vi "Start Sync.vi"(8 "error in (no error)":errorcluster, 11 "gRPC Server in":refnum<class "Data Marshal Server.lvclass">) -> (0 "error out":errorcluster, 3 "gRPC Server out":refnum<class "Data Marshal Server.lvclass">)   [LabVIEW 2019, in "Data Marshal Server.lvlib" / "Data Marshal Server.lvclass"]
uses:
  Data Marshal Server.lvclass
  RPC Messages/TestDataTypesParameters/TestDataTypesParameters_Data.ctl
  RPC Messages/DataTypeTest/DataTypeTest_Data.ctl
  gRPC lvSupport/Server API/typeDefs/grpcId.ctl
  Data Marshal Server.lvclass/Data Marshal Server.ctl
  RPC Messages/ServerEvent/ServerEvent_Data.ctl
  RPC Messages/InvokeResponse/InvokeResponse_Data.ctl
  RPC Messages/QueryResponse/QueryResponse_Data.ctl
  gRPC lvSupport/gprc-lvsupport.lvlib
panel:
  out "Message Data":T1
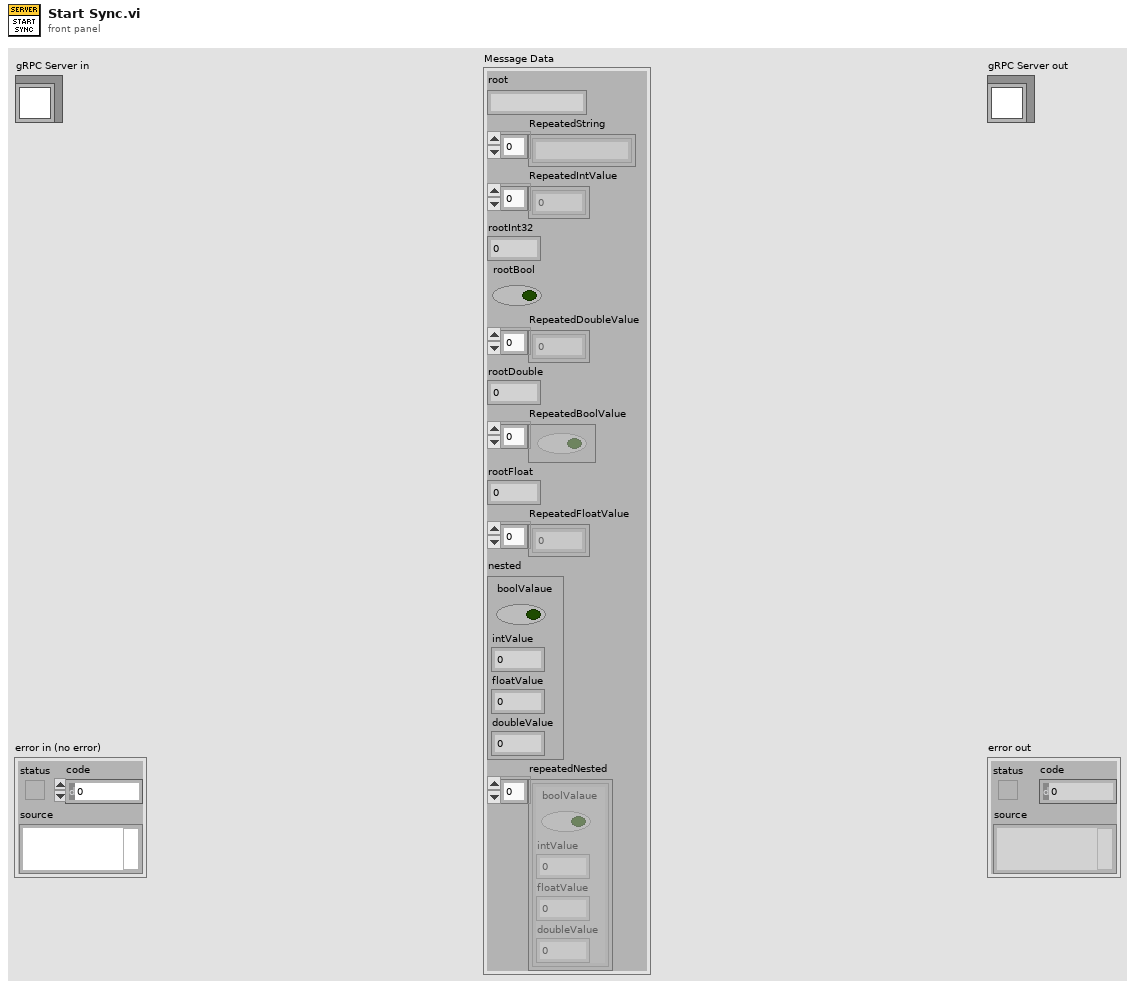
[diagram p1: front panel]
types:
  T1 = typedef "Data Marshal Server.lvlib/Data Marshal Server.lvclass/TestDataTypesParameters_Data.ctl" = cluster{"root":string, "RepeatedString":string[], "RepeatedIntValue":i32[], "rootInt32":i32, "rootBool":bool, "RepeatedDoubleValue":dbl[], "rootDouble":dbl, "RepeatedBoolValue":bool[], "rootFloat":sgl, "RepeatedFloatValue":sgl[], "nested":T2, "repeatedNested":T2[]}
  T2 = typedef "Data Marshal Server.lvlib/Data Marshal Server.lvclass/DataTypeTest_Data.ctl" = cluster{"boolValaue":bool, "intValue":i32, "floatValue":sgl, "doubleValue":dbl}
  T3 = typedef "Data Marshal Server.lvlib/gprc-lvsupport.lvlib/grpcId.ctl" = u64
  T4 = typedef "Data Marshal Server.lvlib/Data Marshal Server.lvclass/ServerEvent_Data.ctl" = cluster{"eventData":string, "serverId":i32, "status":i32}
  T5 = typedef "Data Marshal Server.lvlib/Data Marshal Server.lvclass/InvokeResponse_Data.ctl" = cluster{"status":i32}
  T6 = typedef "Data Marshal Server.lvlib/Data Marshal Server.lvclass/QueryResponse_Data.ctl" = cluster{"message":string, "status":i32}
  T7 = typedef "Data Marshal Server.lvlib/Data Marshal Server.lvclass/Server gRPC UEs.ctl" = cluster{"Invoke gRPC UE":refnum<user-event>, "Query gRPC UE":refnum<user-event>, "Register gRPC UE":refnum<user-event>, "TestDataTypes gRPC UE":refnum<user-event>}
  T8 = typedef "Data Marshal Server.lvlib/Data Marshal Server.lvclass/InvokeRequest_Data.ctl" = cluster{"command":string, "parameter":string}
  T9 = typedef "Data Marshal Server.lvlib/Data Marshal Server.lvclass/QueryRequest_Data.ctl" = cluster{"query":string}
  T10 = typedef "Data Marshal Server.lvlib/Data Marshal Server.lvclass/RegistrationRequest_Data.ctl" = cluster{"eventName":string}
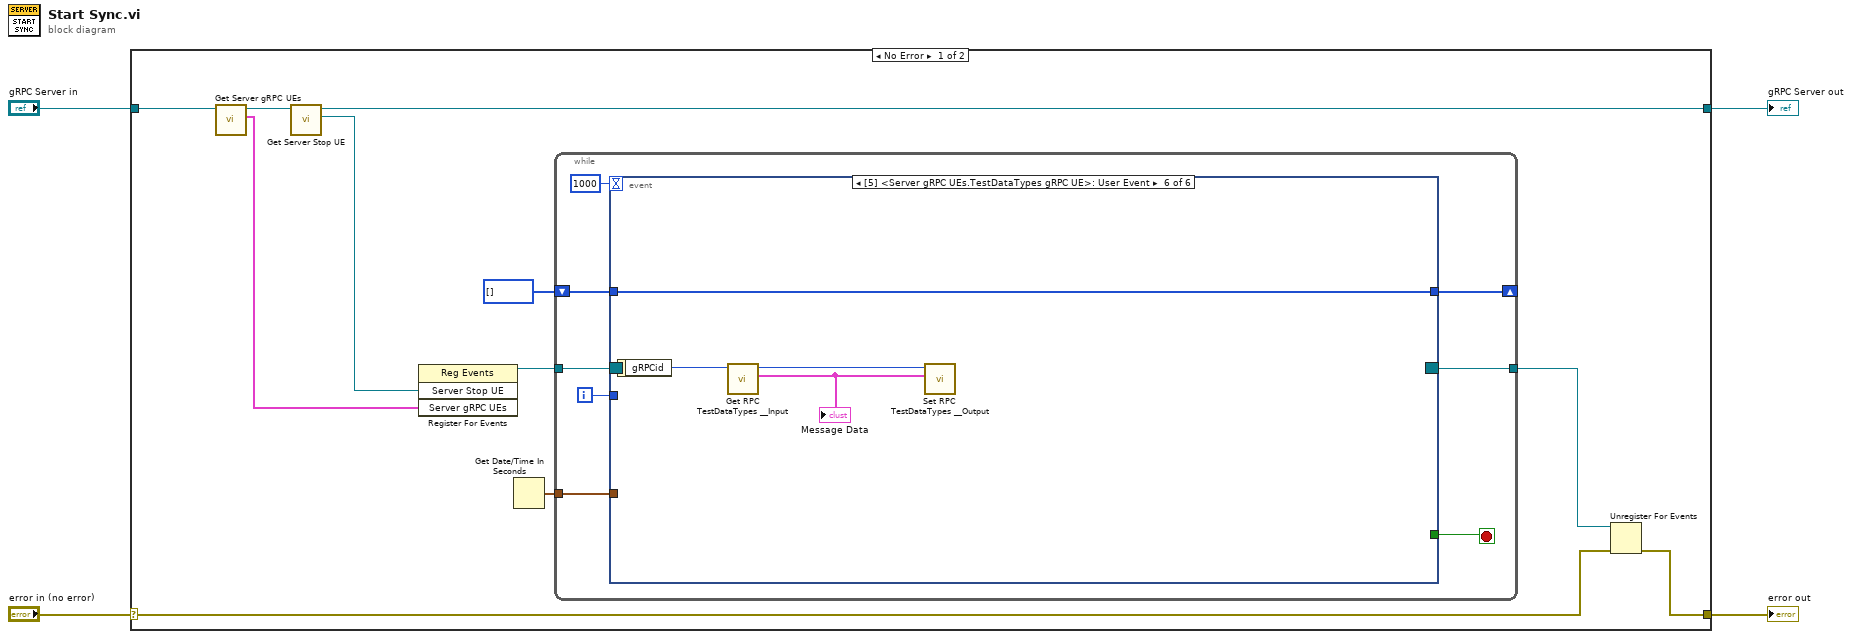
[diagram p0: block diagram]
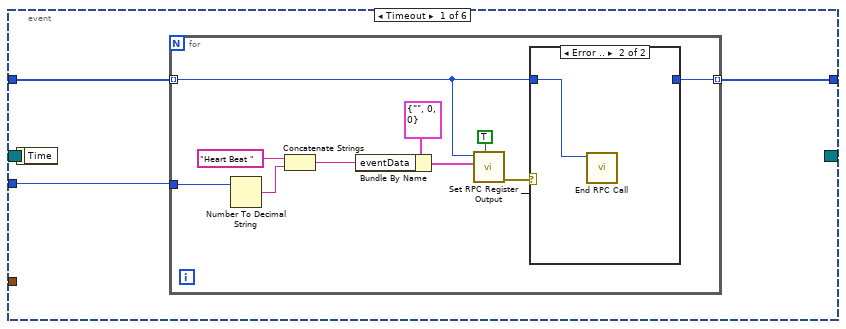
[diagram p2: hidden frame]
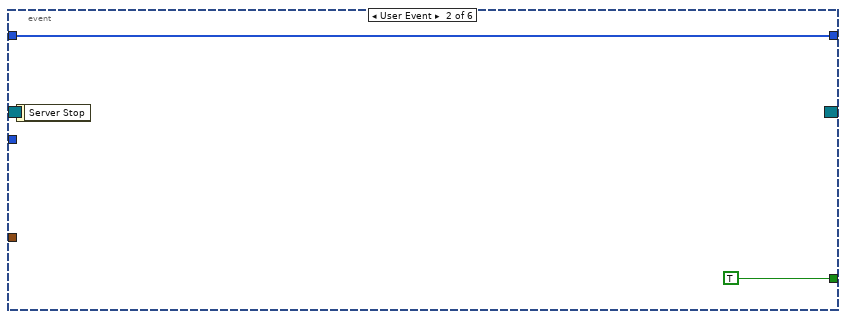
[diagram p4: hidden frame]
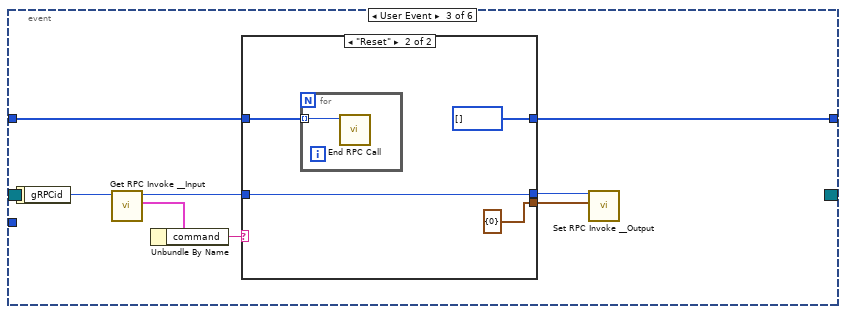
[diagram p5: hidden frame]
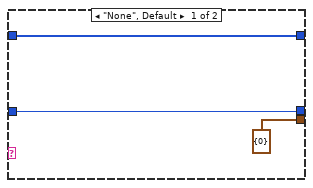
[diagram p6: hidden frame]
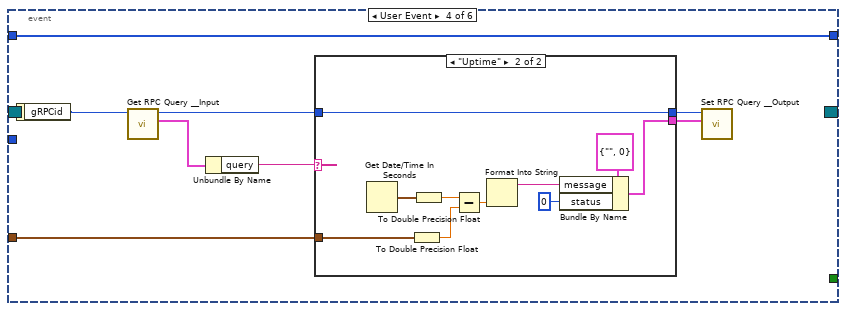
[diagram p7: hidden frame]
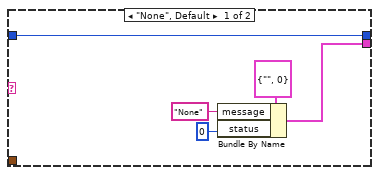
[diagram p8: hidden frame]
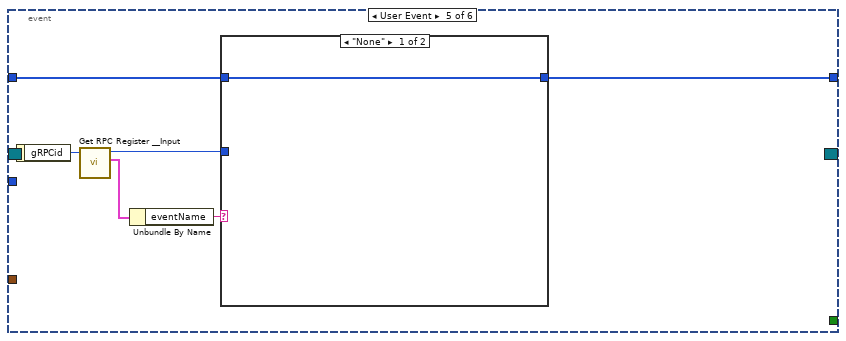
[diagram p9: hidden frame]
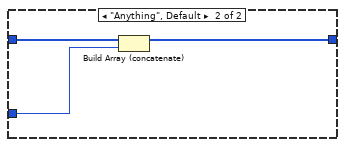
[diagram p10: hidden frame]
diagram:
  n1 = case shown="No Error" "error in (no error)" {
    selector: "error in (no error)" -> [w8 w95]
    tunnel: [w7 w95] -> w3
    tunnel: [w11 w94] -> w1
    tunnel: "gRPC Server in" -> [w15 w94]
    frame No Error {
      n2 = call "Get Server gRPC UEs.vi"("OOP Server in"=w15) -> ("Server gRPC UEs"=w12:T7, "OOP Server out"=w14:refnum<class "Data Marshal Server.lvclass">)  [unwired: 9 in]
      n3 = call "Get Server Stop UE.vi"("OOP Server in"=w14) -> ("Server Stop UE"=w13:refnum<user-event>, "OOP Server out"=w11:refnum<class "Data Marshal Server.lvclass">)  [unwired: 9 in]
      n4 = register-events(w13, w12) -> (reference out=w10:refnum<event-registration>)  [unwired: 2 in, 1 out]
      n5 = Get Date/Time In Seconds() -> (seconds since 1Jan1904=w5:timestamp)
      n6 = while {
        tunnel: w10 -> [w23]
        tunnel: [w21] -> w9
        shift-right: [w18] -> _
        shift-left: T3[] [] ("appended array") -> [w19]
        tunnel: w5 -> [w16]
        i -> [w17]
        stop <- w22 stop-if-true
        n7 = event "RPC Methods Event Structure" shown="[5] <Server gRPC UEs.TestDataTypes gRPC UE>: User Event" {
          selector: w23 -> [_ _ _ _ _ _]
          dyn-events: [_ _ _ _ _ _] -> w21
          timeout: 1000 -> [_ _ _ _ _ _]
          tunnel: [_ TRUE _ _ _ _] -> w22
          tunnel: w19 -> [w26 w39 w45 w64 w81 w93]
          tunnel: [w25 w39 w44 w64 w80 w93] -> w18
          tunnel: w17 -> [w24 _ _ _ _ _]
          tunnel: w16 -> [_ _ _ w57 _ _]
          event Timeout {
            n8 = event-data() -> ()  [unwired: 1 in, 1 out]
            n9 = for {
              tunnel: w26 -> [w29] mode=indexing
              tunnel: w24 -> [w33]
              tunnel: [w27] -> w25 mode=indexing
              n10 = Number To Decimal String(number=w33) -> (decimal integer string=w36:string)  [unwired: 1 in]
              n11 = Concatenate Strings("Heart Beat " ("eventdata"), w36) -> (w34:string)
              n12 = Bundle By Name(cluster=T4 {"eventData"="", "serverId"=0, "status"=0} ("Message Data"), "eventData"=w34) -> (w30:T4)
              n13 = call "Set RPC Register __Output.vi"("Streeming? (F)"=TRUE, "Message Data"=w30, "gRPCid in"=w29) -> ("error out"=w28:errorcluster)  [unwired: 8 in]
              n14 = case shown="Error .." w28 {
                tunnel: w29 -> [w37 w38]
                tunnel: [w37 _] -> w27
                frame No Error {
                }
                frame Error {
                  n15 = call "End RPC Call.vi"("gRPCid"=w38) -> ()  [unwired: 10 in, 1 out]
                }
              }
            }
          }
          event User Event {
            n16 = event-data() -> ()  [unwired: 1 in, 1 out]
          }
          event User Event {
            n17 = event-data() -> ("gRPCid"=w47:T3)  [unwired: 1 in]
            n18 = call "Get RPC Invoke __Input.vi"("gRPCid in"=w47) -> ("Message Data"=w48:T8, "gRPCid out"=w43:T3)  [unwired: 8 in, 1 out]
            n19 = Unbundle By Name(w48) -> ("command"=w46:string)
            n20 = case shown="\"Reset\"" w46 {
              tunnel: [w50 T3[] []] -> w44
              tunnel: w45 -> [w50 w54]
              tunnel: w43 -> [w51 w53]
              tunnel: [w51 w53] -> w42
              tunnel: [T5 {"status"=0} ("Message Data") T5 {"status"=0} ("Message Data")] -> w41
              frame "None", Default {
              }
              frame "Reset" {
                n21 = for {
                  tunnel: w54 -> [w56] mode=indexing
                  n22 = call "End RPC Call.vi"("gRPCid"=w56) -> ()  [unwired: 10 in, 1 out]
                }
              }
            }
            n23 = call "Set RPC Invoke __Output.vi"("Message Data"=w41, "gRPCid in"=w42) -> ()  [unwired: 9 in, 1 out]
          }
          event User Event {
            n24 = event-data() -> ("gRPCid"=w58:T3)  [unwired: 1 in]
            n25 = call "Get RPC Query __Input.vi"("gRPCid in"=w58) -> ("Message Data"=w63:T9, "gRPCid out"=w61:T3)  [unwired: 8 in, 1 out]
            n26 = Unbundle By Name(w63) -> ("query"=w62:string)
            n27 = case shown="\"Uptime\"" w62 {
              tunnel: w61 -> [w65 w79]
              tunnel: [w65 w79] -> w60
              tunnel: [w66 w75] -> w59
              tunnel: w57 -> [_ w72]
              frame "None", Default {
                n28 = Bundle By Name(cluster=T6 {"message"="", "status"=0} ("Message Data"), "message"="None", "status"=0) -> (w66:T6)
              }
              frame "Uptime" {
                n29 = Get Date/Time In Seconds() -> (seconds since 1Jan1904=w74:timestamp)
                n30 = To Double Precision Float(number=w72) -> (double precision float=w71:dbl)
                n31 = To Double Precision Float(number=w74) -> (double precision float=w73:dbl)
                n32 = Subtract(x=w73, y=w71) -> (x-y=w78:dbl)
                n33 = Format Into String(w78) -> (resulting string=w76:string)  [unwired: 3 in, 1 out]
                n34 = Bundle By Name(cluster=T6 {"message"="", "status"=0} ("Message Data"), "message"=w76, "status"=0) -> (w75:T6)
              }
            }
            n35 = call "Set RPC Query __Output.vi"("Message Data"=w59, "gRPCid in"=w60) -> ()  [unwired: 9 in, 1 out]
          }
          event User Event {
            n36 = event-data() -> ("gRPCid"=w85:T3)  [unwired: 1 in]
            n37 = call "Get RPC Register __Input.vi"("gRPCid in"=w85) -> ("Message Data"=w84:T10, "gRPCid out"=w82:T3)  [unwired: 8 in, 1 out]
            n38 = Unbundle By Name(w84) -> ("eventName"=w83:string)
            n39 = case shown="\"None\"" w83 {
              tunnel: w82 -> [_ w89]
              tunnel: w81 -> [w86 w88]
              tunnel: [w86 w87] -> w80
              frame "None" {
              }
              frame "Anything", Default {
                n40 = Build Array (concatenate)(w88, w89) -> (w87:T3[])
              }
            }
          }
          event User Event {
            n41 = event-data() -> ("gRPCid"=w90:T3)  [unwired: 1 in]
            n42 = call "Get RPC TestDataTypes __Input.vi"("gRPCid in"=w90) -> ("Message Data"=w91:T1, "gRPCid out"=w92:T3)  [unwired: 8 in, 1 out]
            "Message Data" <- w91
            n43 = call "Set RPC TestDataTypes __Output.vi"("Message Data"=w91, "gRPCid in"=w92) -> ()  [unwired: 9 in, 1 out]
          }
        }
      }
      n44 = Unregister For Events(event registration refnum=w9, error in=w8) -> (error out=w7:errorcluster)
    }
    frame Error {
    }
  }
  "error out" <- w3
  "gRPC Server out" <- w1
